vi "Get Wafer ID.vi"(8 "error in (no error)":errorcluster, 11 "VISA resource name":refnum<visa-resource-name>="GPIB1::11::INSTR") -> (0 "error out":errorcluster, 2 "Wafer_ID":string)   [LabVIEW 2013]
uses:
  Public/Documents/National Instruments/TestStand 2013/Components/Modules/NI_SemiconductorModule/Handlers/TEL_P-8_P-12XL/Source/TEL GPIB Command Set/TEL GPIB Command Set.lvlib
panel:
  out "return count":u32
  # "GR11608-E5"
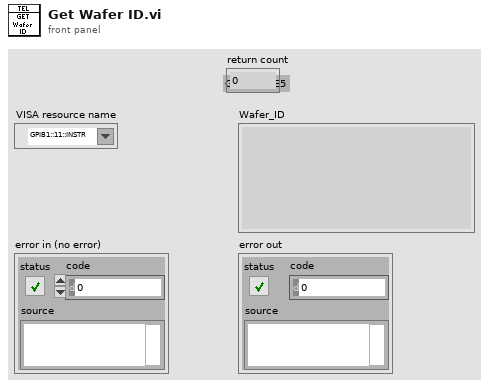
[diagram p1: front panel]
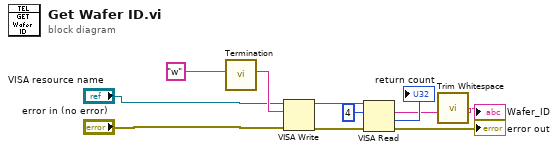
[diagram p0: block diagram]
diagram:
  n1 = call "Termination.vi"("Input"="w" ("string")) -> ("Output"=w10:string)  [unwired: 10 in]
  n2 = VISA Write(VISA resource name="VISA resource name", write buffer=w10, error in (no error)="error in (no error)") -> (VISA resource name out=w9:refnum<visa-resource-name>, error out=w8:errorcluster)  [unwired: 1 out]
  n3 = VISA Read(VISA resource name=w9, byte count=u32 4, error in (no error)=w8) -> (read buffer=w2:string, return count=→"return count":u32, error out=→"error out":errorcluster)  [unwired: 1 out]
  n4 = call <vilib>:"Trim Whitespace.vi"("string"=w2) -> ("trimmed string"=→"Wafer_ID":string)  [unwired: 1 in]
